vi "add_std_data.vi"(0 "Analysis in":refnum<class "Analysis.lvclass">, 5 "standard_name":string, 7 "standard_type":string, 9 "Isotope Table":cluster{"isotope":string, "amount cc":dbl}[](array[cluster]), 11 "error in (no error)":errorcluster) -> (4 "Analysis out":refnum<class "Analysis.lvclass">, 15 "error out":errorcluster)   [LabVIEW 2017]
doc: "Reformats the standard data and saves them in the StandardDataArray of the AnalysisObject"
uses:
  Analysis.lvclass
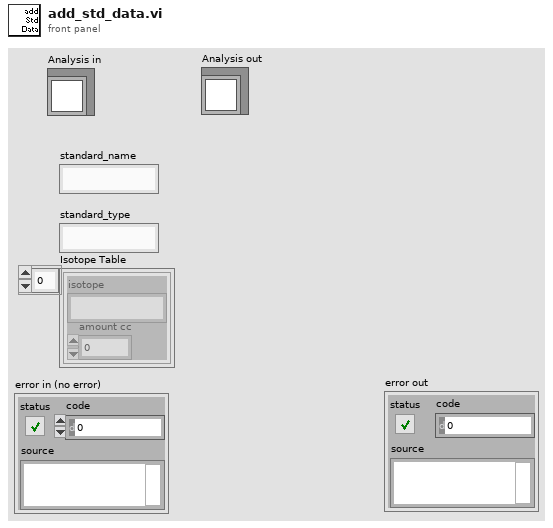
[diagram p1: front panel]
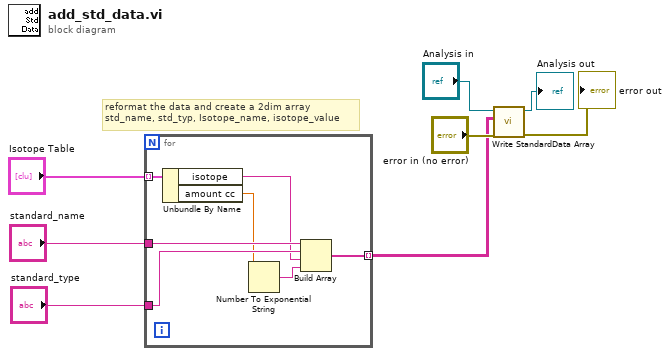
[diagram p0: block diagram]
diagram:
  # "reformat the data and create a 2dim array\nstd_name, std_typ, Isotope_name, isotope_value"
  n1 = for {
    tunnel: "Isotope Table" -> [w13] mode=indexing
    tunnel: "standard_name" -> [w15]
    tunnel: "standard_type" -> [w14]
    tunnel: [w9] -> w5 mode=indexing
    n2 = Unbundle By Name(w13) -> ("isotope"=w12:string, "amount cc"=w10:dbl)
    n3 = Number To Exponential String(number=w10) -> (E-format string=w11:string)  [unwired: 3 in]
    n4 = Build Array(w15, w14, w12, w11) -> (w9:string[])
  }
  n5 = call-dynamic "Write StandardData Array.vi"("error in (no error)"="error in (no error)", "StandardData Array"=w5, "Analysis in"="Analysis in") -> ("error out"=→"error out":errorcluster, "Analysis out"=→"Analysis out":refnum<class "Analysis.lvclass">)  [unwired: 7 in]
